vi "Create Network Stream Initiator.vi"(6 "Buffer Size":i32=4096, 8 "Remote Context":string, 9 "Remote Name":string, 10 "Remote Address":string, 11 "Name":string) -> (3 "Network Stream Initiator out":refnum<class "Network Stream Initiator.lvclass">)   [LabVIEW 2020, in "Network Stream Initiator.lvclass"]
doc: "Use this method to configure a Network Stream Initiator with connection information for its remote counterpart."
uses:
  <vilib>/NI/Actors/Network Endpoint Actors/Protocols/Network Stream Strategy/Network Stream Initiator/Network Stream Initiator.lvclass
  C:/Program Files (x86)/National Instruments/LabVIEW 2020/vi.lib/NI/Actors/Network Endpoint Actors/Protocols/Network Stream Strategy/Network Stream/Network Stream.lvclass
  <vilib>/NI/Actors/Network Endpoint Actors/Protocols/Network Stream Strategy/Network Stream/Network Stream.lvclass/Network Stream.ctl
  <vilib>/NI/Actors/Network Endpoint Actors/Protocols/Network Stream Strategy/Network Stream Initiator/Network Stream Initiator.lvclass/Network Stream Initiator.ctl
  <vilib>/NI/Actors/Network Endpoint Actors/Protocols/Network Stream Strategy/Network Stream/Network Stream.lvclass
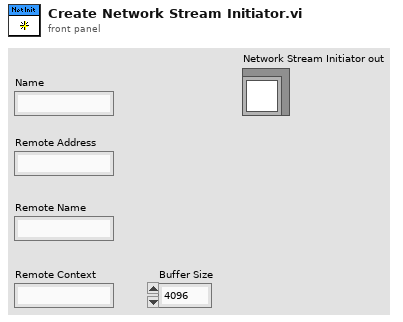
[diagram p1: front panel]
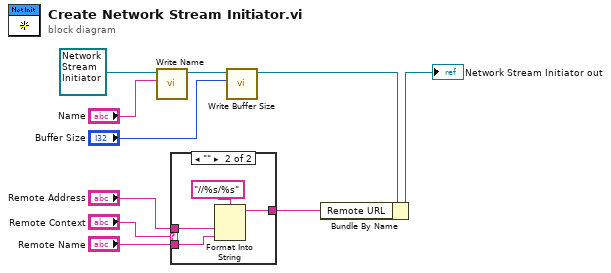
[diagram p0: block diagram]
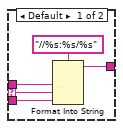
[diagram p2: hidden frame]
diagram:
  n1 = call <vilib>:"Write Name.vi"("Name"="Name", "Network Stream in"=refnum<class "Network Stream Initiator.lvclass"> refnum ("Network Stream Initiator in")) -> ("Network Stream out"=w4:refnum<class "Network Stream Initiator.lvclass">)  [unwired: 9 in]
  n2 = case shown="\"\"" "Remote Context" {
    selector: "Remote Context" -> [w12 _]
    tunnel: [w14 w18] -> w6
    tunnel: "Remote Name" -> [w13 w17]
    tunnel: "Remote Address" -> [w11 w16]
    frame Default {
      n3 = Format Into String(format string="//%s:%s/%s", w11, w12, w13) -> (resulting string=w14:string)  [unwired: 2 in, 1 out]
    }
    frame "" {
      n4 = Format Into String(format string="//%s/%s", w16, w17) -> (resulting string=w18:string)  [unwired: 2 in, 1 out]
    }
  }
  n5 = call <vilib>:"Write Buffer Size.vi"("Buffer Size"="Buffer Size", "Network Stream in"=w4) -> ("Network Stream out"=w3:refnum<class "Network Stream Initiator.lvclass">)  [unwired: 9 in]
  n6 = Bundle By Name(cluster=w3, "Remote URL"=w6) -> (→"Network Stream Initiator out":refnum<class "Network Stream Initiator.lvclass">)
